vi "Read Matlab Params.vi"(8 "error in (no error)":errorcluster, 10 "Enum":T1(ring), 11 "TrialBasedExperiment in":refnum<class "ClassDiscrimination.lvclass">) -> (0 "error out":errorcluster, 2 "Matlab Param Array":cluster{"Name":string, "Data":variant}[](array[cluster]), 3 "TrialBasedExperiment out":refnum<class "ClassDiscrimination.lvclass">)   [LabVIEW 2011, in "ClassDiscrimination.lvclass"]
uses:
  ClassDiscrimination.lvclass
  Trial Based Experiment Statechart/MatlabExperiment/MatlabExperiment.lvclass
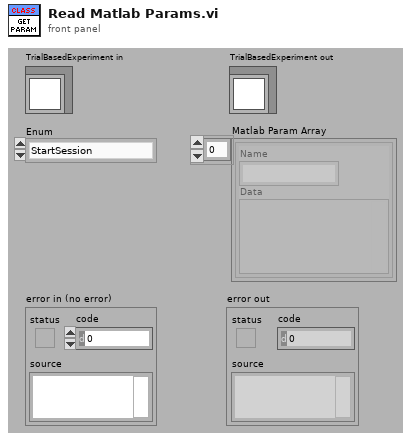
[diagram p1: front panel]
types:
  T1 = enum16{"StartSession", "StartTrial", "ShowStimulus"}
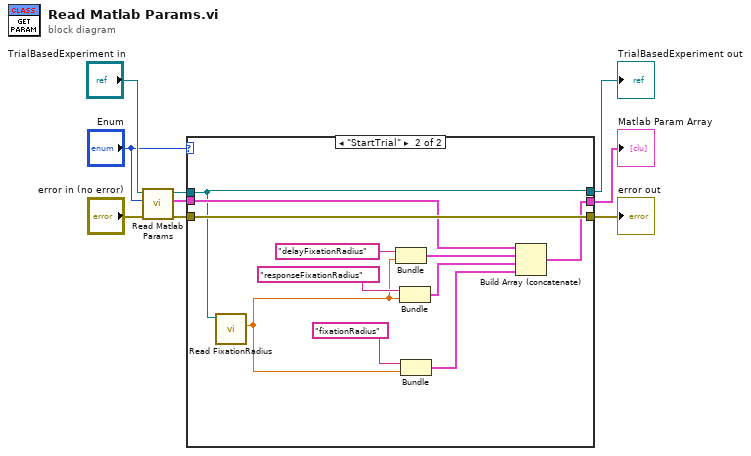
[diagram p0: block diagram]
diagram:
  n1 = call-parent "Read Matlab Params.vi"("error in (no error)"="error in (no error)", "Enum"="Enum", "TrialBasedExperiment in"="TrialBasedExperiment in") -> ("error out"=w5:errorcluster, "Matlab Param Array"=w4:cluster{"Name":string, "Data":variant}[], "TrialBasedExperiment out"=w6:refnum<class "ClassDiscrimination.lvclass">)  [unwired: 6 in]
  n2 = case shown="\"StartTrial\"" "Enum" {
    tunnel: w6 -> [w12 w15]
    tunnel: w5 -> [w11 w23]
    tunnel: [w12 w15] -> w2
    tunnel: w4 -> [w10 w21]
    tunnel: [w11 w23] -> w3
    tunnel: [w10 w19] -> w1
    frame "StartSession", Default {
    }
    frame "StartTrial" {
      n3 = call-dynamic "Read FixationRadius.vi"("MatlabExperiment in"=w15) -> ("FixationRadius"=w14:dbl)  [unwired: 8 in, 2 out]
      n4 = Bundle("delayFixationRadius", "FixationRadius"=w14) -> (w20:cluster{string, "FixationRadius":dbl})  [unwired: 1 out]
      n5 = Bundle("responseFixationRadius", "FixationRadius"=w14) -> (w17:cluster{string, "FixationRadius":dbl})  [unwired: 1 out]
      n6 = Bundle("fixationRadius", "FixationRadius"=w14) -> (w13:cluster{string, "FixationRadius":dbl})  [unwired: 1 out]
      n7 = Build Array (concatenate)(w21, w20, w17, w13) -> (w19:cluster{"Name":string, "Data":variant}[])
    }
  }
  "error out" <- w3
  "TrialBasedExperiment out" <- w2
  "Matlab Param Array" <- w1
